vi "BLOW.vi"(10 "argv":string[](array[string]), 11 "args":u8) -> ()   [LabVIEW 2011]
uses:
  roller/roller_user_state.ctl
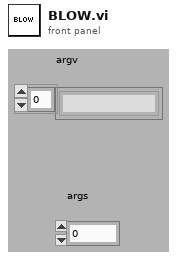
[diagram p1: front panel]
types:
  T1 = typedef "roller_user_state.ctl" = enum16{"off", "collect", "blow", "force suck"}
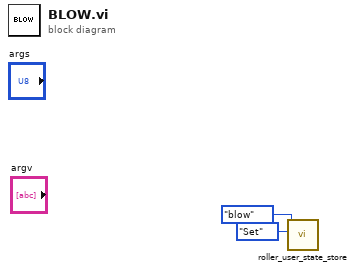
[diagram p0: block diagram]
diagram:
  n1 = call "roller_user_state_store.vi"("data_store_mode"=enum16{"Set", "Get"}."Set", "roller user state"=roller_user_state."blow") -> ()  [unwired: 9 in, 1 out]
